vi "Seq Motor Dialog Teach.vi"(8 "Segment Data":T1) -> (0 "Step Hisitory":string[](array[string]), 2 "Segment Data 2":T1)   [LabVIEW 2015]
uses:
  Sequence/type defs/Sequence Info.ctl
  type defs/Motor Teach.ctl
panel:
  in  "Current threshold":dbl
  in  "Detection time":u32
  out "String 2":string="Pre Run Station - Glass - Vent Open"
  out "error out":errorcluster
  in  "Description":string
  in  "Save":bool
  in  "Cancel":bool
  # "ms"
  # "A"
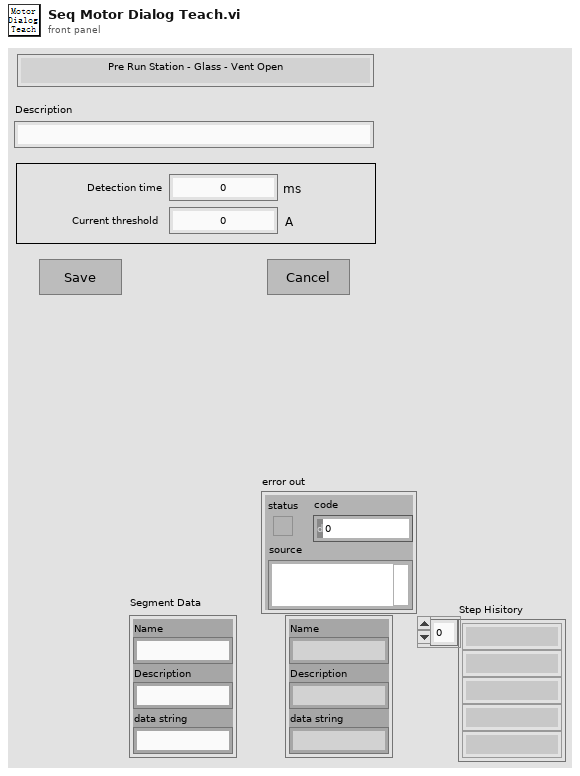
[diagram p1: front panel]
types:
  T1 = typedef "Sequence Info.ctl" = cluster{"Name":string, "Description":string, "data string":string}
  T2 = typedef "Motor Teach.ctl" = cluster{"Current threshold":dbl, "Detection time":u32}
  T3 = cluster{"Segment Data":T1, "Motor Teach":T2, "Old Data":string, "New Data":string}
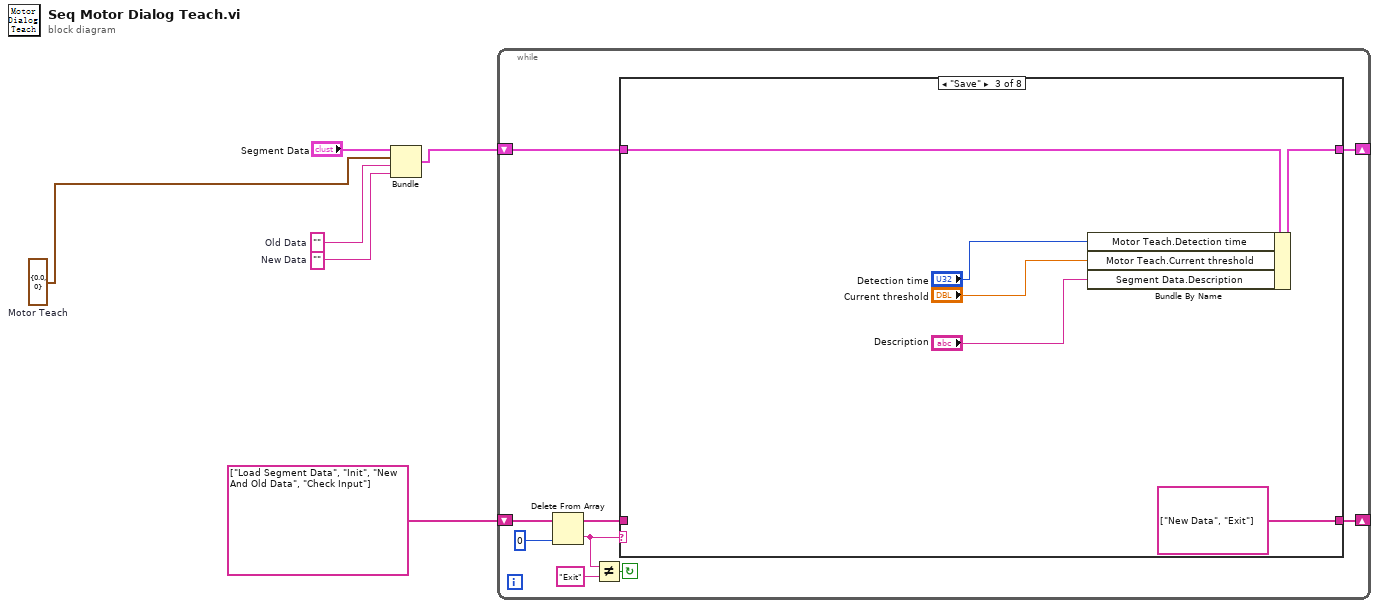
[diagram p0: block diagram]
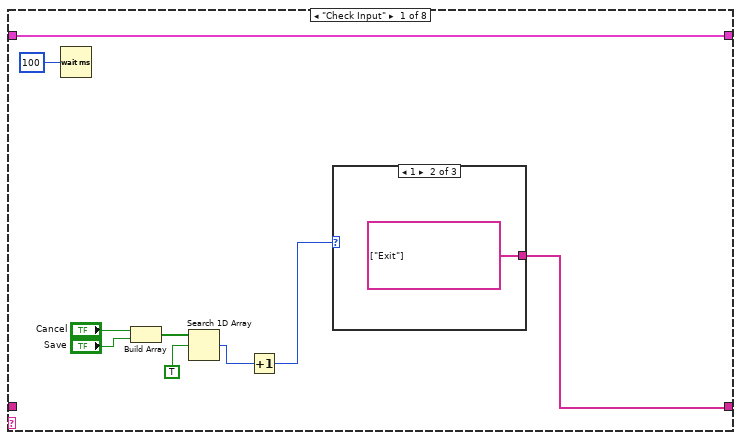
[diagram p2: hidden frame]
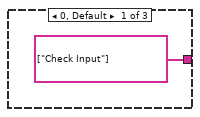
[diagram p3: hidden frame]
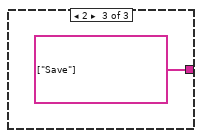
[diagram p4: hidden frame]
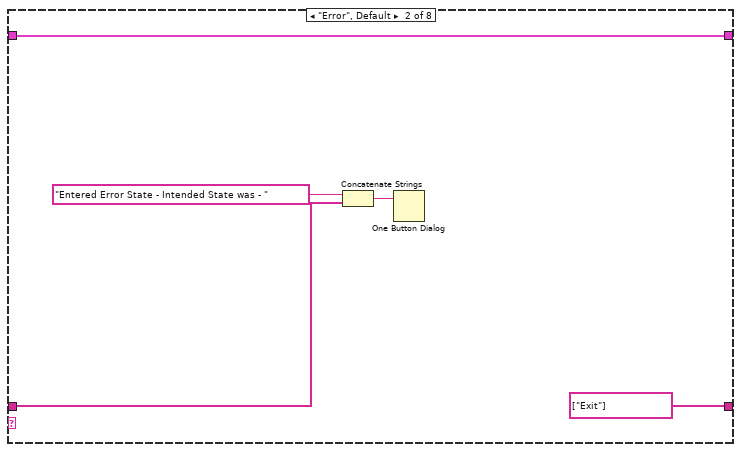
[diagram p5: hidden frame]
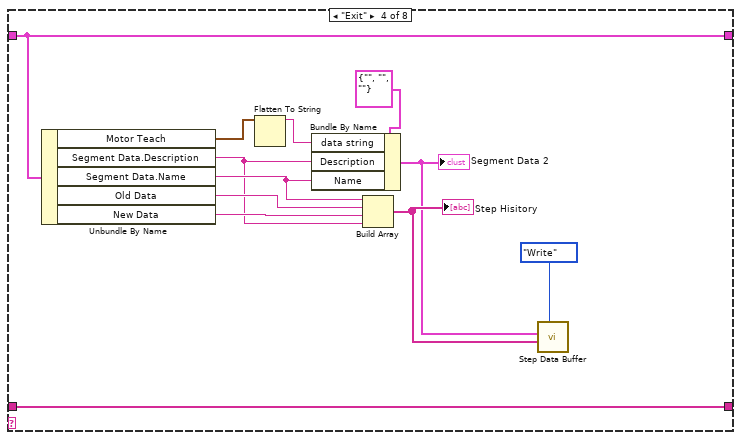
[diagram p6: hidden frame]
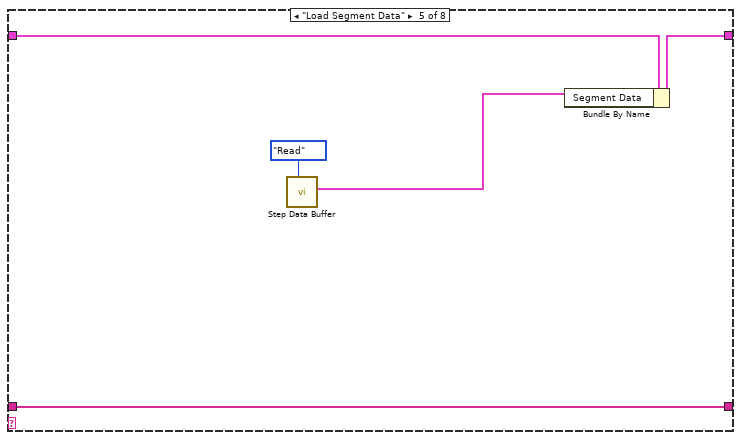
[diagram p7: hidden frame]
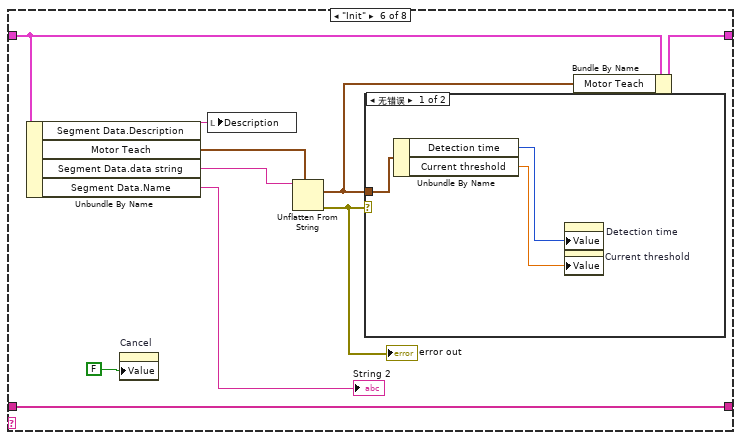
[diagram p8: hidden frame]
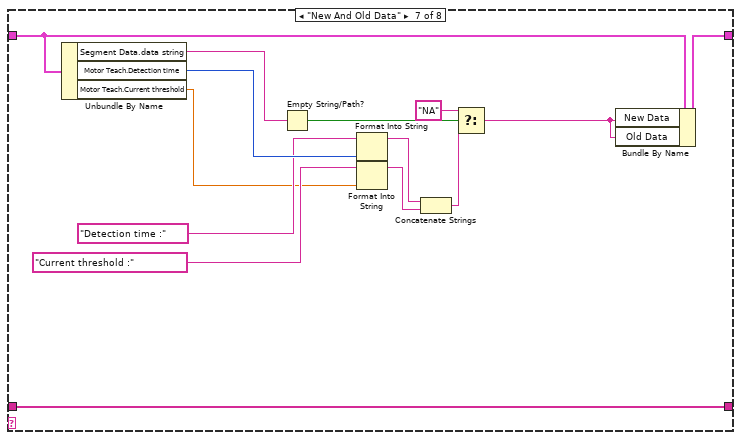
[diagram p10: hidden frame]
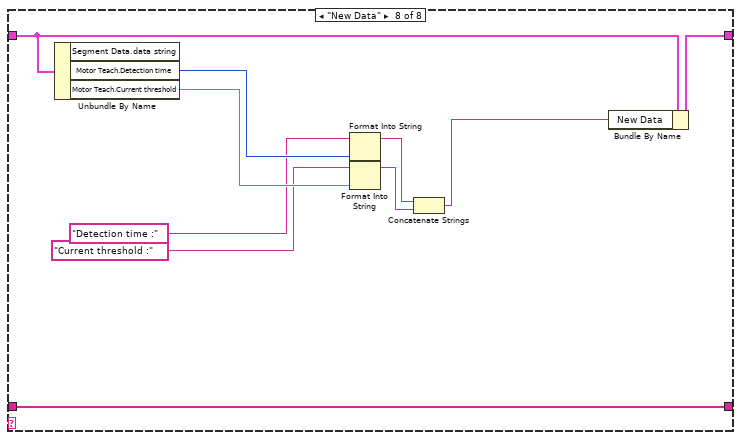
[diagram p11: hidden frame]
diagram:
  w1 = T2 {"Current threshold"=0.0, "Detection time"=0}  # Motor Teach
  w3 = ""  # New Data
  w4 = ""  # Old Data
  n1 = Bundle("Segment Data"="Segment Data", "Motor Teach"=w1, "Old Data"=w4, "New Data"=w3) -> (w5:T3)  [unwired: 1 in]
  n2 = while {
    shift-right: [w15] -> _
    shift-left: string[] ["Load Segment Data", "Init", "New And Old Data", "Check Input"] ("Event queue out") -> [w11]
    shift-right: [w13] -> _
    shift-left: w5 -> [w14]
    stop <- w7 continue-if-true
    n3 = Delete From Array(array=w11, index=0 ("Index")) -> (deleted portion=w9:string, array with subset deleted=w10:string[])  [unwired: 1 in]
    n4 = Not Equal?(x=w9, y="Exit" ("Exit Event")) -> (x != y?=w7:bool)
    n5 = case shown="\"Save\"" w9 {
      tunnel: w10 -> [_ w29 _ w50 w55 w65 w82 w86]
      tunnel: [w16 string[] ["Exit"] ("event queue out") string[] ["New Data", "Exit"] ("Event queue out") w50 w55 w65 w82 w86] -> w15
      tunnel: w14 -> [w19 w32 w37 w43 w52 w58 w71 w85]
      tunnel: [w19 w32 w36 w43 w51 w57 w70 w84] -> w13
      frame "Check Input" {
        n6 = Wait (ms)(milliseconds to wait=u32 100) -> ()  [unwired: 1 out]
        n7 = Build Array("Cancel", "Save") -> (w21:bool[])
        n8 = Search 1D Array(1D array=w21, element=TRUE) -> (index of element=w17:i32)  [unwired: 1 in]
        n9 = Increment(x=w17) -> (x+1=w18:i32)
        n10 = case shown="1" w18 {
          tunnel: [string[] ["Check Input"] ("Events to Insert") string[] ["Exit"] ("Events to Insert") string[] ["Save"] ("Events to Insert")] -> w16
          frame 0, Default {
          }
          frame 1 {
          }
          frame 2 {
          }
        }
      }
      frame "Error", Default {
        n11 = Concatenate Strings("Entered Error State - Intended State was - " ("string"), w29) -> (w30:string)
        n12 = One Button Dialog(message=w30) -> ()  [unwired: 1 in, 1 out]
      }
      frame "Save" {
        n13 = Bundle By Name(cluster=w37, "Motor Teach.Detection time"="Detection time", "Motor Teach.Current threshold"="Current threshold", "Segment Data.Description"="Description") -> (w36:T3)
      }
      frame "Exit" {
        n14 = Unbundle By Name(w43) -> ("Motor Teach"=w49:T2, "Segment Data.Description"=w39:string, "Segment Data.Name"=w44:string, "Old Data"=w46:string, "New Data"=w45:string)
        n15 = Flatten To String(anything=w49) -> (data string=w47:string)  [unwired: 3 in, 2 out]
        n16 = Bundle By Name(cluster=T1 {"Name"="", "Description"="", "data string"=""} ("Segment Data"), "data string"=w47, "Description"=w39, "Name"=w44) -> (w40:T1)
        "Segment Data 2" <- w40
        n17 = Build Array(w44, w46, w45, w39) -> (w41:string[])
        "Step Hisitory" <- w41
        n18 = call "Step Data Buffer.vi"("Mode"=enum16{"Init", "Read", "Write"}."Write", "Step Hisitory In"=w41, "Segment Data"=w40) -> ()  [unwired: 4 in, 5 out]
      }
      frame "Load Segment Data" {
        n19 = call "Step Data Buffer.vi"("Mode"=enum16{"Init", "Read", "Write"}."Read") -> ("Segment Data"=w53:T1)  [unwired: 6 in, 4 out]
        n20 = Bundle By Name(cluster=w52, "Segment Data"=w53) -> (w51:T3)
      }
      frame "Init" {
        n21 = Unbundle By Name(w58) -> ("Segment Data.Description"=w60:string, "Motor Teach"=w63:T2, "Segment Data.data string"=w64:string, "Segment Data.Name"=→"String 2":string)
        n22 = property on="Cancel" class="Bool (严格)"("Value"=FALSE ("Cancel")) -> ()  [unwired: 2 in, 2 out]
        n23 = local write "Description"(w60) -> ()
        n24 = Unflatten From String(type=w63, binary string=w64) -> (value=w59:T2, error out=w62:errorcluster)  [unwired: 3 in, 1 out]
        "error out" <- w62
        n25 = case shown="无错误" w62 {
          tunnel: w59 -> [w68 _]
          frame No Error {
            n26 = Unbundle By Name(w68) -> ("Detection time"=w67:u32, "Current threshold"=w66:dbl)
            n27 = property on="Detection time" class="DigNum (严格)"("Value"=w67) -> ()  [unwired: 2 in, 2 out]
            n28 = property on="Current threshold" class="DigNum (严格)"("Value"=w66) -> ()  [unwired: 2 in, 2 out]
          }
          frame Error {
          }
        }
        n29 = Bundle By Name(cluster=w58, "Motor Teach"=w59) -> (w57:T3)
      }
      frame "New And Old Data" {
        n30 = Unbundle By Name(w71) -> ("Segment Data.data string"=w81:string, "Motor Teach.Detection time"=w76:u32, "Motor Teach.Current threshold"=w69:dbl)
        n31 = Empty String/Path?(string/path=w81) -> (empty?=w80:bool)
        n32 = Format Into String(initial string="Detection time :" ("string"), w76) -> (resulting string=w75:string)  [unwired: 2 in, 1 out]
        n33 = Format Into String(initial string="Current threshold :" ("string"), w69) -> (resulting string=w74:string)  [unwired: 2 in, 1 out]
        n34 = Concatenate Strings(w75, w74) -> (w77:string)
        n35 = Select(t="NA", s=w80, f=w77) -> (s? t:f=w78:string)
        n36 = Bundle By Name(cluster=w71, "New Data"=w78, "Old Data"=w78) -> (w70:T3)
      }
      frame "New Data" {
        n37 = Unbundle By Name(w85) -> ("Motor Teach.Detection time"=w92:u32, "Motor Teach.Current threshold"=w90:dbl)  [unwired: 1 out]
        n38 = Format Into String(initial string="Detection time :" ("string"), w92) -> (resulting string=w91:string)  [unwired: 2 in, 1 out]
        n39 = Format Into String(initial string="Current threshold :" ("string"), w90) -> (resulting string=w89:string)  [unwired: 2 in, 1 out]
        n40 = Concatenate Strings(w91, w89) -> (w83:string)
        n41 = Bundle By Name(cluster=w85, "New Data"=w83) -> (w84:T3)
      }
    }
  }
